vi "Transceiver.Command.Send.vi"(8 "error in (no error)":errorcluster, 9 "timeout in ms (0)":i32 format="%d ms", 10 "command":T1={"Command"=enum."Rx", "Command Parameters"={"arg1"=0, "arg2"=0}}, 11 "Transceiver Interface in":refnum<class "Transceiver Interface.lvclass">) -> (0 "error out":errorcluster, 1 "timed out?":bool, 3 "Transceiver Interface out":refnum<class "Transceiver Interface.lvclass">)   [LabVIEW 2017, in "DSF.Engine.lvlib" / "Transceiver Thread.lvclass"]
uses:
  Transceiver Thread.lvclass
  Interface/Transceiver Interface.lvclass
  C:/Git/DSF/DSF Core/Source/Engine/Classes/Interface/Interface.lvclass
  Interface/Transceiver Interface.Command Data.ctl
  Interface/Transceiver Interface.Command.ctl
  Interface/Transceiver Interface.Command Parameters.ctl
  Interface/Interface.lvclass/Interface.ctl
  Debug/FIFO Flags.lvclass/FIFO Flags.ctl
  Interface/Transceiver Interface.Write.Command.vi
  Interface/Interface.Write.Command.vi
  Interface/Interface.Get Command FIFO.vi
  Interface/Interface.RT FIFO.Write.16B.vi
  Interface/Interface.Get Debug Flags.vi
  Debug/FIFO Flags.Get Infinite Timeouts.vi
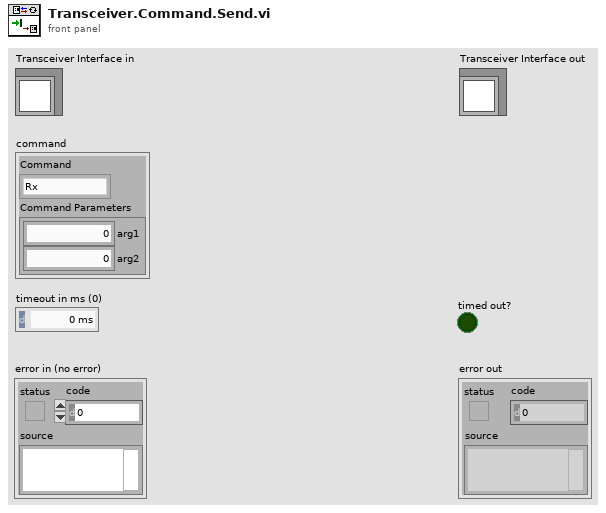
[diagram p1: front panel]
types:
  T1 = typedef "DSF.Engine.lvlib/Transceiver Interface.lvclass/Transceiver Interface.Command Data.ctl" = cluster{"Command":T2, "Command Parameters":T3}
  T2 = typedef "DSF.Engine.lvlib/Transceiver Interface.lvclass/Transceiver Interface.Command.ctl" = enum8{"Set Base Pointer", "Rx", "Tx", "Shutdown"}
  T3 = typedef "DSF.Engine.lvlib/Transceiver Interface.lvclass/Transceiver Interface.Command Parameters.ctl" = cluster{"arg1":u64, "arg2":u64}
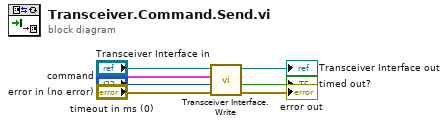
[diagram p0: block diagram]
diagram:
  n1 = call-poly "Transceiver Interface.Write.vi"("error in (no error)"="error in (no error)", "timeout in ms (0)"="timeout in ms (0)", "command"="command", "Transceiver Interface in"="Transceiver Interface in") -> ("error out"=→"error out":errorcluster, "timed out?"=→"timed out?":bool, "Transceiver Interface out"=→"Transceiver Interface out":refnum<class "Transceiver Interface.lvclass">)  [unwired: 5 in]
